vi "APC_9049_9056SharedVarPolling.vi"(0 "Number of signals":i32) -> (1 "Number of signals (out)":i32, 2 "TimeStamp9056":dbl, 3 "9056 IO":dbl[](array[numeric]), 4 "SystemState":dbl)   [LabVIEW 2020]
doc: "This example demonstrates the procedure required to apply different NI-DAQmx Custom Scales to each virtual channel in a task. A DAQmx Task Property Node (Functions >> NI Measurements >> DAQmx - Data Acquisition >> DAQmx Advanced Task Options) is used to obtain the task's virtual channels. A DAQmx Channel Property Node (Functions >> NI Measurements >> DAQmx - Data Acquisition) is then used to set the custom scale for each virtual channel in the task.\n\nThe \"DAQmx Create Scale\" VI creates a custom scale for each channel in the channel list. *Note, make sure your Minimum and Maximum channel parameters are consistent with the range the scale will create."
panel:
  out "error out":errorcluster
  out "9056_raster":string[](array[string])
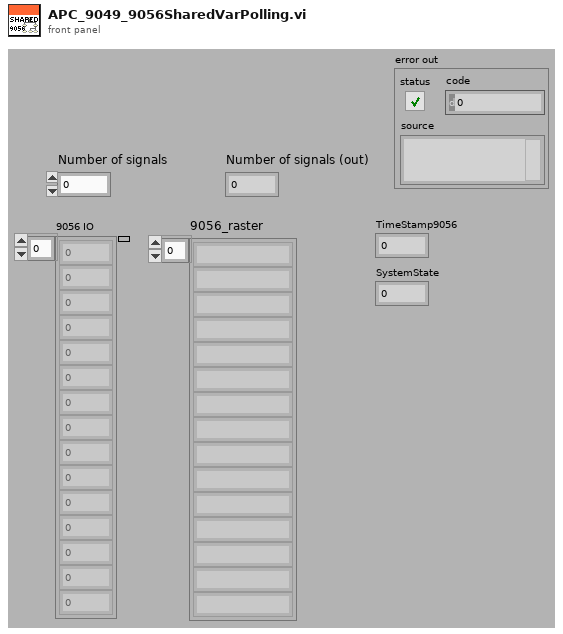
[diagram p1: front panel]
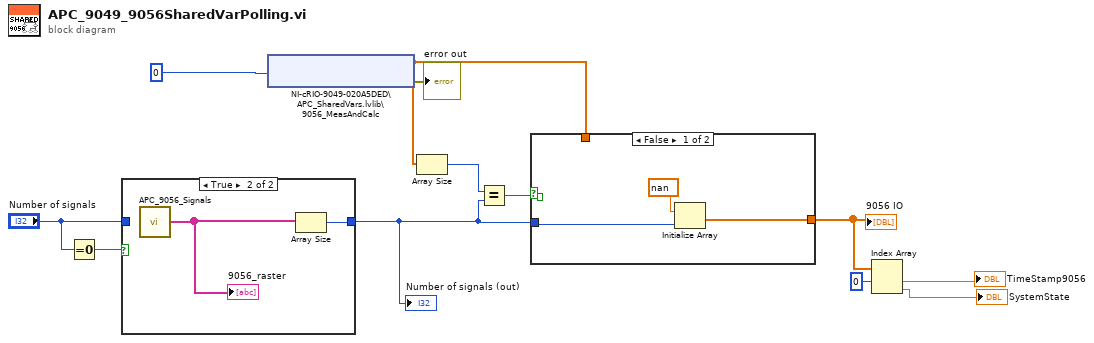
[diagram p0: block diagram]
diagram:
  n1 = Equal To 0?(x="Number of signals") -> (x = 0?=w10:bool)
  n2 = case shown="True" w10 {
    tunnel: [w13 w15] -> w8
    tunnel: "Number of signals" -> [w13 _]
    frame False {
    }
    frame True {
      n3 = call "APC_9056_Signals.vi"() -> ("9056_raster"=w14:string[])  [unwired: 3 in, 2 out]
      "9056_raster" <- w14
      n4 = Array Size(array=w14) -> (size(s)=w15:i32)
    }
  }
  "Number of signals (out)" <- w8
  n5 = shared-variable "NI-cRIO-9049-020A5DED\\APC_SharedVars.lvlib\\9056_MeasAndCalc"(0 ("ms timeout (0)")) -> (w7:dbl[], error out=→"error out":errorcluster)  [unwired: 1 in, 1 out]
  n6 = Array Size(array=w7) -> (size(s)=w12:i32)
  n7 = Equal?(x=w12, y=w8) -> (x = y?=w11:bool)
  n8 = case shown="False" w11 {
    tunnel: w7 -> [_ w19]
    tunnel: w8 -> [w18 _]
    tunnel: [w16 w19] -> w4
    frame False {
      n9 = Initialize Array(nan ("element"), w18) -> (w16:dbl[])
    }
    frame True {
    }
  }
  "9056 IO" <- w4
  n10 = Index Array(array=w4, index #1=0 ("index")) -> (element #1=→"TimeStamp9056":dbl, element #2=→"SystemState":dbl)  [unwired: 1 in]
